vi "Set Scale (SubVI).vi"(2 "error in":errorcluster, 3 "Scale":i32=999, 4 "VISA Refnum in":refnum<visa-resource-name>) -> (0 "error out":errorcluster, 1 "VISA Refnum out":refnum<visa-resource-name>)   [LabVIEW 2017]
doc: "by Tanguy BOULARD"
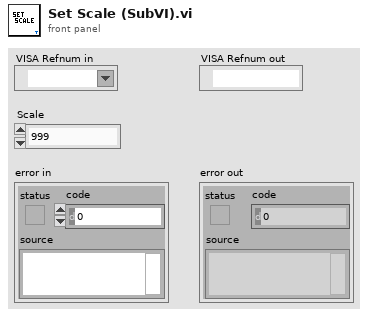
[diagram p1: front panel]
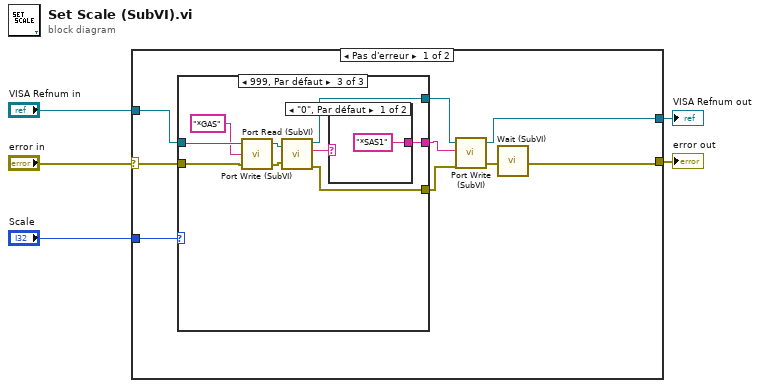
[diagram p0: block diagram]
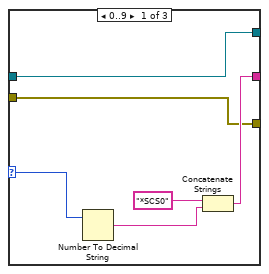
[diagram p2: hidden frame]
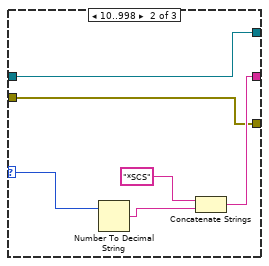
[diagram p3: hidden frame]
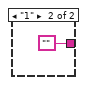
[diagram p4: hidden frame]
diagram:
  n1 = case shown="Pas d'erreur" "error in" {
    selector: "error in" -> [w12 w39]
    tunnel: [w9 w39] -> w4
    tunnel: "VISA Refnum in" -> [w11 w38]
    tunnel: [w8 w38] -> w2
    tunnel: "Scale" -> [w13 _]
    frame No Error {
      n2 = case shown="999, Par défaut" w13 {
        selector: w13 -> [w20 w25 _]
        tunnel: w12 -> [w16 w22 w35]
        tunnel: w11 -> [w15 w21 w28]
        tunnel: [w17 w23 w31] -> w6
        tunnel: [w16 w22 w30] -> w10
        tunnel: [w15 w21 w29] -> w7
        frame 0..9 {
          n3 = Number To Decimal String(number=w20) -> (decimal integer string=w18:string)  [unwired: 1 in]
          n4 = Concatenate Strings("*SCS0" ("format string"), w18) -> (w17:string)
        }
        frame 10..998 {
          n5 = Number To Decimal String(number=w25) -> (decimal integer string=w24:string)  [unwired: 1 in]
          n6 = Concatenate Strings("*SCS" ("format string"), w24) -> (w23:string)
        }
        frame 999, Default {
          n7 = call "Port Write (SubVI).vi"("error in"=w35, "write buffer"="*GAS", "VISA Refnum in"=w28) -> ("error out"=w33:errorcluster, "VISA Refnum out"=w34:refnum<visa-resource-name>)  [unwired: 1 in]
          n8 = call "Port Read (SubVI).vi"("VISA Refnum in"=w34, "error in"=w33) -> ("VISA Refnum out"=w29:refnum<visa-resource-name>, "chaîne concaténée"=w32:string, "error out"=w30:errorcluster)  [unwired: 1 out]
          n9 = case shown="\"0\", Par défaut" w32 {
            tunnel: ["*SAS1" ""] -> w31
            frame "0", Default {
            }
            frame "1" {
            }
          }
        }
      }
      n10 = call "Port Write (SubVI).vi"("error in"=w10, "write buffer"=w6, "VISA Refnum in"=w7) -> ("error out"=w14:errorcluster, "VISA Refnum out"=w8:refnum<visa-resource-name>)  [unwired: 1 in]
      n11 = call "Wait (SubVI).vi"("error in"=w14) -> ("error out"=w9:errorcluster)  [unwired: 26 in]
    }
    frame Error {
    }
  }
  "error out" <- w4
  "VISA Refnum out" <- w2
